vi "Generate Transfer Function.vi"(8 "Error In":errorcluster, 11 "Mode In":refnum<class "Mode.lvclass">) -> (0 "Error Out":errorcluster, 3 "Mode Out":refnum<class "Mode.lvclass">)   [LabVIEW 2023, in "Mode.lvclass"]
uses:
  Mode.lvclass
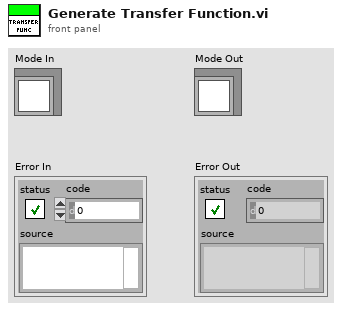
[diagram p1: front panel]
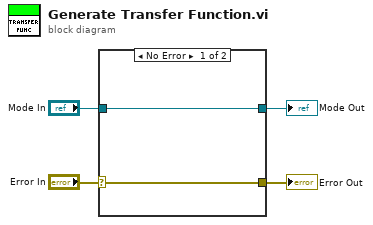
[diagram p0: block diagram]
diagram:
  n1 = case shown="No Error" "Error In" {
    selector: "Error In" -> [w5 w8]
    tunnel: [w5 w8] -> w3
    tunnel: [w6 w7] -> w1
    tunnel: "Mode In" -> [w6 w7]
    frame No Error {
    }
    frame Error {
    }
  }
  "Error Out" <- w3
  "Mode Out" <- w1
